vi "Improved population speed.vi"() -> ()   [LabVIEW 2018]
panel:
  in  "Userfiles Directory":path=path "C:/Projects/SmartGrid/ICDAS/UserFiles-PMU"
  in  "Tree":string(tree)
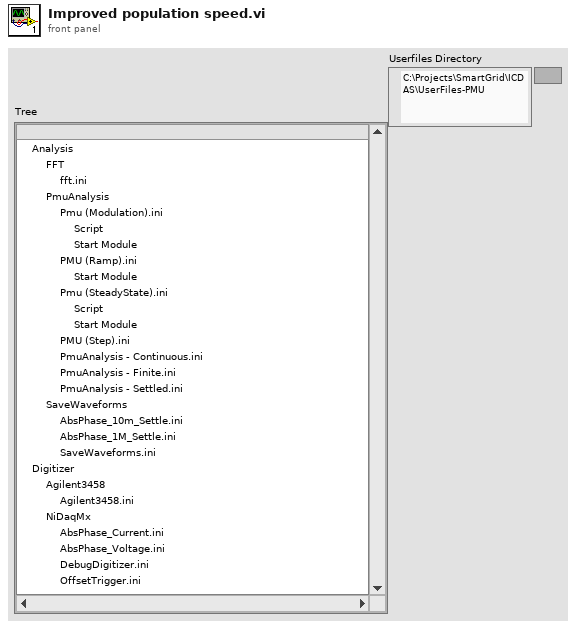
[diagram p1: front panel]
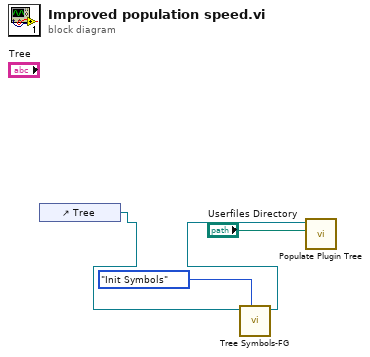
[diagram p0: block diagram]
diagram:
  n1 = control-ref of="Tree"() -> (w2:refnum<vi>)
  n2 = call "Tree Symbols-FG.vi"("Actions"=enum16{"Init Symbols", "Set Item Symbol"}."Init Symbols", "Tree Ref"=w2) -> ("Tree Ref out"=w1:refnum<vi>)  [unwired: 7 in, 2 out]
  n3 = call "Populate Plugin Tree.vi"("Userfiles Directory"="Userfiles Directory", "PluginTreeRef"=w1) -> ()  [unwired: 7 in, 3 out]
